vi "Write Test Case object to front panel control.vi"(8 "error in (no error)":errorcluster, 10 "VI Refnum":refnum<vi>, 11 "Test Case in":refnum<class "LUnit Test Case V2.lvclass">) -> (0 "error out":errorcluster, 2 "VI Refnum out":refnum<vi>, 3 "Test Case out":refnum<class "LUnit Test Case V2.lvclass">)   [LabVIEW 2020, in "LUnit Test Case V2.lvclass"]
uses:
  LUnit Test Case V2.lvclass
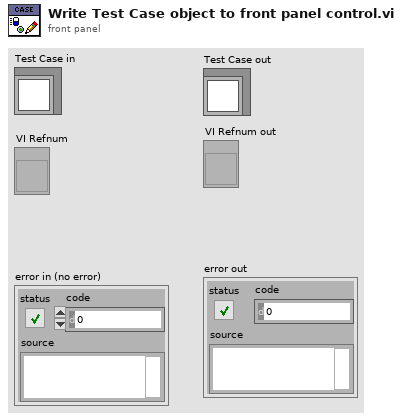
[diagram p1: front panel]
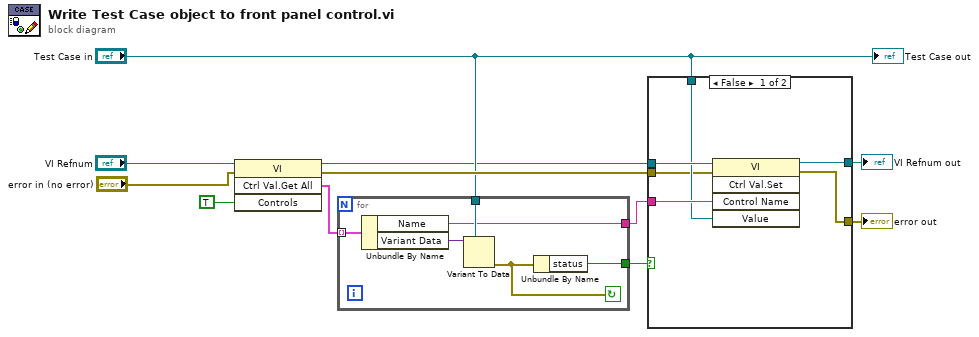
[diagram p0: block diagram]
diagram:
  n1 = invoke on="Invoke Node" class="VI" method="Ctrl Val.Get All"(reference="VI Refnum", error in="error in (no error)", "Controls"=TRUE) -> (reference out=w4:refnum<vi>, error out=w10:errorcluster, "Get All Control Values Variant"=w6:cluster{"Name":string, "Variant Data":variant}[])  [unwired: 1 in, 1 out]
  n2 = for {
    tunnel: w6 -> [w17] mode=indexing
    tunnel: "Test Case in" -> [w15]
    tunnel: [w14] -> w7
    tunnel: [w12] -> w8
    stop <- w13 continue-if-true
    n3 = Unbundle By Name(w17) -> ("Name"=w14:string, "Variant Data"=w16:variant)
    n4 = Variant To Data(type=w15, Variant=w16) -> (error out=w13:errorcluster)  [unwired: 1 in, 1 out]
    n5 = Unbundle By Name(w13) -> ("status"=w12:bool)
  }
  n6 = case shown="False" w8 {
    tunnel: w4 -> [w23 w25]
    tunnel: w7 -> [w22 _]
    tunnel: "Test Case in" -> [w21 _]
    tunnel: w10 -> [w20 w24]
    tunnel: [w19 w25] -> w2
    tunnel: [w18 w24] -> w1
    frame False {
      n7 = invoke on="Invoke Node" class="VI" method="Ctrl Val.Set"(reference=w23, error in=w20, "Control Name"=w22, "Value"=w21) -> (reference out=w19:refnum<vi>, error out=w18:errorcluster)  [unwired: 1 in, 3 out]
    }
    frame True {
    }
  }
  "VI Refnum out" <- w2
  "error out" <- w1
  "Test Case out" <- "Test Case in"
